vi "PicoScope3000aExampleBlock.vi"() -> ()   [LabVIEW 2018]
panel:
  in  "Trigger Settings":T1={"Trigger Enabled"=FALSE, "Trigger Source"=enum."Channel A", "Trigger Threshold (volts)"=0.0, "Trigger Direction"=2, "Trigger Delay (samples)"=0, "Auto Trigger Time (ms)"=1000} {"Trigger Direction" items=["Above", "Below", "Rising", "Falling", "Rising or Falling"]}
  in  "Channel A Settings":T2={"Enabled"=TRUE, "Coupling"=1, "Range"=6, "Analogue Offset"=0.0} {"Range" items=["10 mV", "20 mV", "50 mV", "100 mV", "200 mV", "500 mV", "1 V", "2 V", "5 V", "10 V", "20 V", "50 V ", "100 V"]; "Coupling" items=["AC", "DC"]}
  out "USB 3.0 device on non-USB 3.0 Port":bool=TRUE
  out "USB Powered":bool=TRUE
  in  "Acquisition Settings":T3={"preTriggerSamples"=0, "postTriggerSamples"=1000, "timebase"=2, "Down-Sample Mode"=0, "Down Sample Ratio"=1} {"Down Sample Ratio" min=1 step=1; "Down-Sample Mode" items=["None"=0, "Aggregate"=1, "Decimate"=2, "Average"=4]}
  out "Channel A":T4(graph)
  out "Device Info":T5
  in  "Use Serial number":bool
  in  "Batch/Serial":string
  out "Properties Panel":T6 {"Max Total Capture Time Available (sec)" format="%.3p"; "Sample Frequency" format="%.3p"; "Sample Rate" format="%.3p"; "Max Samples Available" format="%.3p"; "Total Capture Time (sec)" format="%.3p"}
  in  "stop":bool
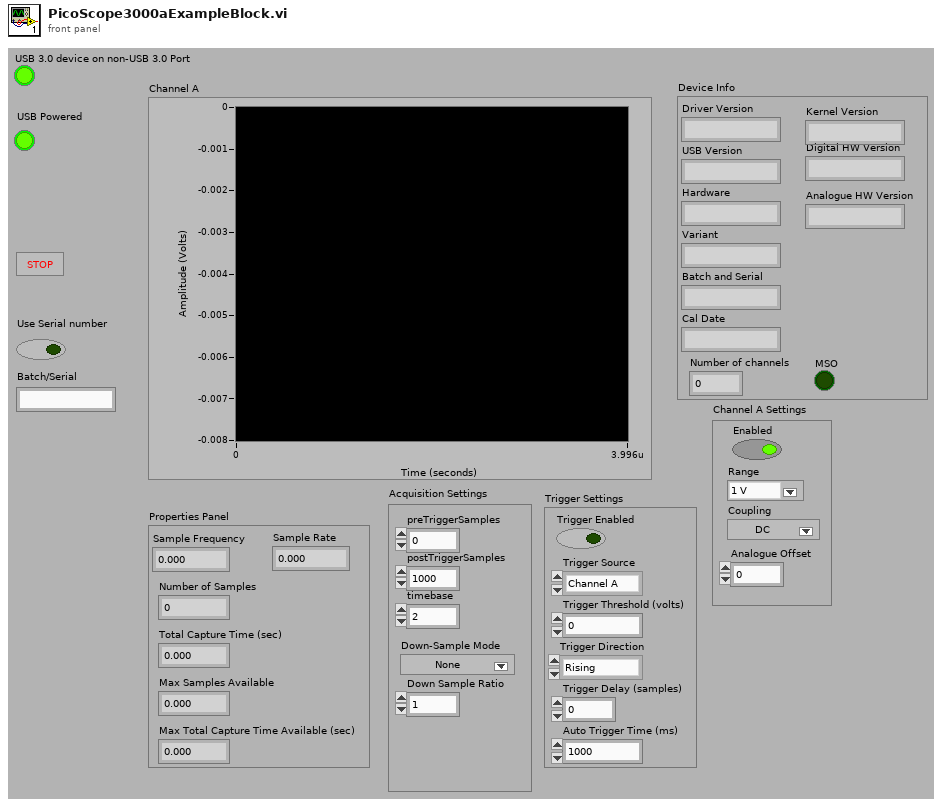
[diagram p1: front panel]
types:
  T1 = cluster{"Trigger Enabled":bool, "Trigger Source":enum32{"Channel A", "Channel B", "Channel C", "Channel D", "Ext."}, "Trigger Threshold (volts)":dbl, "Trigger Direction":u16, "Trigger Delay (samples)":u32, "Auto Trigger Time (ms)":i16}
  T2 = cluster{"Enabled":bool, "Coupling":u32, "Range":u32, "Analogue Offset":sgl}
  T3 = cluster{"preTriggerSamples":u32, "postTriggerSamples":u32, "timebase":u32, "Down-Sample Mode":i32, "Down Sample Ratio":u32}
  T4 = cluster{i32, "Sample Rate":sgl, "Data (Volts)":dbl[]}
  T5 = cluster{"Driver Version":string, "USB Version":string, "Hardware":string, "Variant":string, "Batch and Serial":string, "Cal Date":string, "Kernel Version":string, "Digital HW Version":string, "Analogue HW Version":string, "MSO":bool, "Number of channels":i16}
  T6 = cluster{"Sample Frequency":sgl, "Sample Rate":sgl, "Max Samples Available":i32, "Number of Samples":u32, "Total Capture Time (sec) ":sgl, "Max Total Capture Time Available (sec)":sgl}
  T7 = cluster{"Channel D Buffer":i16[], "Channel C Buffer":i16[], "Channel B Buffer":i16[], "Channel A Buffer":i16[], "Port 0  Buffer ":i16[], "Port 1 Buffer ":i16[]}
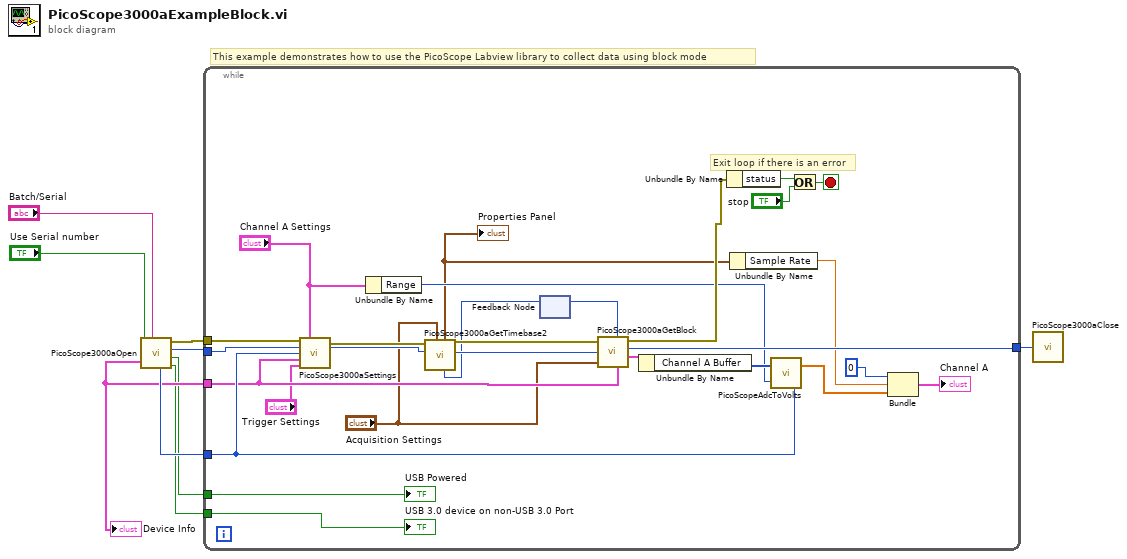
[diagram p0: block diagram]
diagram:
  # "This example demonstrates how to use the PicoScope Labview library to collect data using block mode"
  n1 = call "PicoScope3000aOpen.vi"("Batch/Serial"="Batch/Serial", "Use Serial number"="Use Serial number") -> ("USB 3.0 device on non-USB 3.0 Port"=w1:bool, "USB Powered"=w2:bool, "handle"=w7:i16, "error out"=w8:errorcluster, "Max ADC value"=w4:i16, "Device Info"=w3:T5)  [unwired: 4 in]
  "Device Info" <- w3
  n2 = while {
    tunnel: w7 -> [w35]
    tunnel: w8 -> [w34]
    tunnel: [w27] -> w9
    tunnel: w4 -> [w22]
    tunnel: w3 -> [w15]
    tunnel: w2 -> [w13]
    tunnel: w1 -> [w12]
    stop <- w37 stop-if-true
    # "Exit loop if there is an error"
    n3 = call "PicoScope3000aSettings.vi"("error in"=w34, "Channel A Settings"="Channel A Settings", "handle in"=w35, "Max_adc"=w22, "Device Info"=w15, "Trigger Settings"="Trigger Settings") -> ("error out"=w31:errorcluster, "handle out"=w30:i16)  [unwired: 7 in, 1 out]
    n4 = Unbundle By Name("Channel A Settings") -> ("Range"=w21:u32)
    n5 = feedback #1() -> (w24:u32)  [unwired: 1 in]
    n6 = call "PicoScope3000aGetTimebase2.vi"("Number of Samples"=w24, "Acquisition Settings"="Acquisition Settings", "handle in"=w30, "error in (no error)"=w31) -> ("handle out"=w28:i16, "error out"=w29:errorcluster, "Properties Panel"=w17:T6)  [unwired: 5 in]
    "Properties Panel" <- w17
    n7 = call "PicoScope3000aGetBlock.vi"("error in"=w29, "handle in"=w28, "Acquisition Settings"="Acquisition Settings", "Device Info"=w15) -> ("noOfSamples"=w25:u32, "error out"=w26:errorcluster, "handle out"=w27:i16, "Buffers (Max or non-aggregated)"=w33:T7)  [unwired: 1 in, 2 out]
    n8 = feedback-in #1(w25) -> ()
    n9 = Unbundle By Name(w33) -> ("Channel A Buffer"=w23:i16[])
    n10 = Unbundle By Name(w26) -> ("status"=w32:bool)
    n11 = Unbundle By Name(w17) -> ("Sample Rate"=w16:sgl)
    n12 = call "PicoScopeAdcToVolts.vi"("Max_adc"=w22, "Range Index"=w21, "Data"=w23) -> ("Data (Volts)"=w18:dbl[])
    n13 = Or(x=w32, y="stop") -> (x .or. y?=w37:bool)
    n14 = Bundle(0, "Sample Rate"=w16, "Data (Volts)"=w18) -> (→"Channel A":T4)  [unwired: 1 in]
    "USB Powered" <- w13
    "USB 3.0 device on non-USB 3.0 Port" <- w12
  }
  n15 = call "PicoScope3000aClose.vi"("handle"=w9) -> ()
